vi "Update Icon Name.vi"(8 "error in (no error)":errorcluster, 10 "Device Icon Name Array":string[](array[string]), 11 "Device Ref":refnum<data-value>) -> (0 "error out":errorcluster, 3 "Device Ref":refnum<data-value>)   [LabVIEW 2014, in "Device.lvclass"]
uses:
  Device.lvclass
  Device.lvclass/Device.ctl
  Device Configuration/Device Configuration.lvclass/Device Configuration.ctl
  Device Configuration/Device Configuration.lvclass
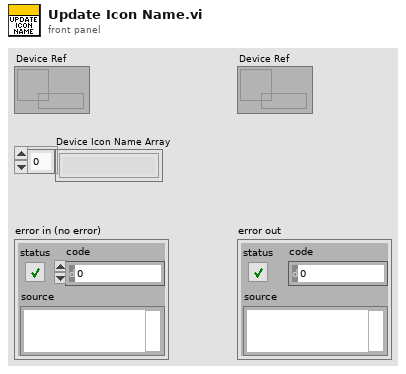
[diagram p1: front panel]
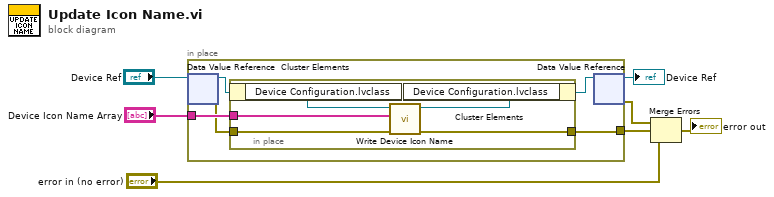
[diagram p0: block diagram]
diagram:
  n1 = in-place {
    in-place-border: "Device Icon Name Array" -> [w10]
    in-place-border: [w8] -> w4
    n2 = in-place-dvr #1("Device Ref") -> (w12:refnum<class "Device.lvclass">, w9:errorcluster)
    n3 = in-place {
      in-place-border: w10 -> [w15]
      in-place-border: w9 -> [w14]
      in-place-border: [w13] -> w8
      n4 = in-place-cluster #2(w12) -> ("Device Configuration.lvclass"=w17:refnum<class "Device Configuration.lvclass">)
      n5 = call "Write Device Icon Name.vi"("error in (no error)"=w14, "Device Icon Name"=w15, "Device Configuration in"=w17) -> ("error out"=w13:errorcluster, "Device Configuration out"=w16:refnum<class "Device Configuration.lvclass">)  [unwired: 7 in]
      n6 = in-place-cluster #2("Device Configuration.lvclass"=w16) -> (w11:refnum<class "Device.lvclass">)
    }
    n7 = in-place-dvr #1(w11) -> (→"Device Ref":refnum<data-value>, w5:errorcluster)
  }
  n8 = Merge Errors(w5, w4, "error in (no error)") -> (→"error out":errorcluster)
